vi "OPVM.vi"() -> ()   [LabVIEW 2013]
uses:
  <instrlib>/Keithley 24XX/Public/Data/Read (Multiple Points).vi
  <instrlib>/Keithley 24XX/Keithley 24XX.lvlib
panel:
  out "Voc":sgl
  out "Log IV Graph":cluster{"Voltage":sgl[], "Current":sgl[]}(graph)
  out "IV Graph":cluster{"Voltage":sgl[], "Current":sgl[]}(graph)
  in  "Source Mode  (0: Voltage)":u16(ring) items=["Voltage", "Current"]
  in  "Serial Configuration":T1={"Baud Rate"=9600, "Parity"=0, "Data Bits"=8, "Stop Bits"=10, "Flow Control"=0} {"Flow Control" items=["None", "XON/XOFF", "RTS/CTS", "XON/XOFF & RTS/CTS", "DTR/DSR", "XON/XOFF & DTR/DSR"]; "Stop Bits" items=["1.0"=10, "1.5"=15, "2.0"=20]; "Data Bits" items=["7"=7, "8"=8]; "Parity" items=["None", "Odd", "Even", "Mark", "Space"]; "Baud Rate" items=["300"=300, "600"=600, "1200"=1200, "2400"=2400, "4800"=4800, "9600"=9600, "19200"=19200]}
  in  "VISA resource name":refnum<visa-resource-name>
  in  "Timeout (10000 ms)":i32=10000 format="%#.6g"
  in  "END":dbl=2.0
  in  "START":dbl=1.0
  in  "Number of Points (5)":u32=5
  in  "Current Range (compliance)":dbl=0.1
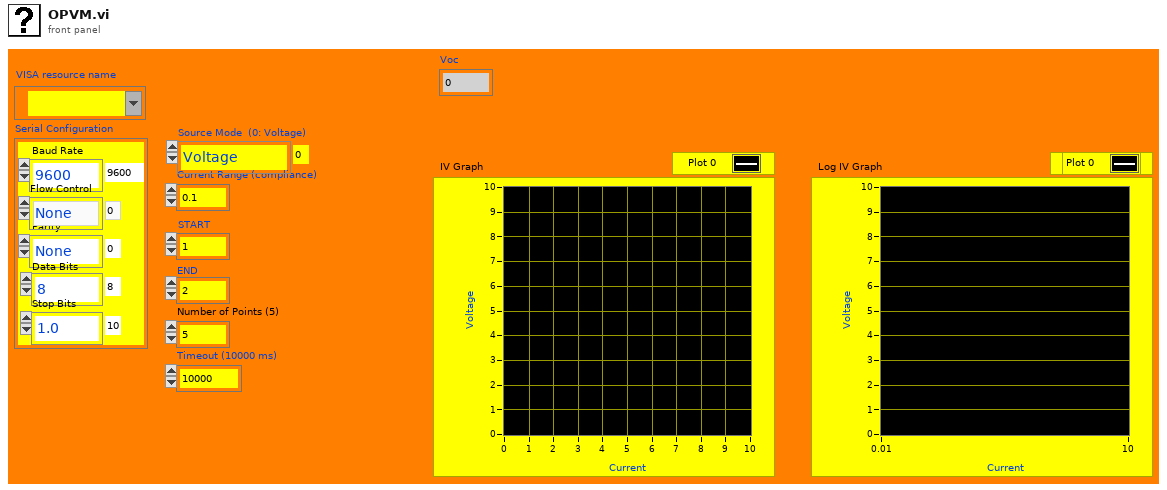
[diagram p1: front panel]
types:
  T1 = cluster{"Baud Rate":u32, "Parity":u16, "Data Bits":u16, "Stop Bits":u16, "Flow Control":u16}
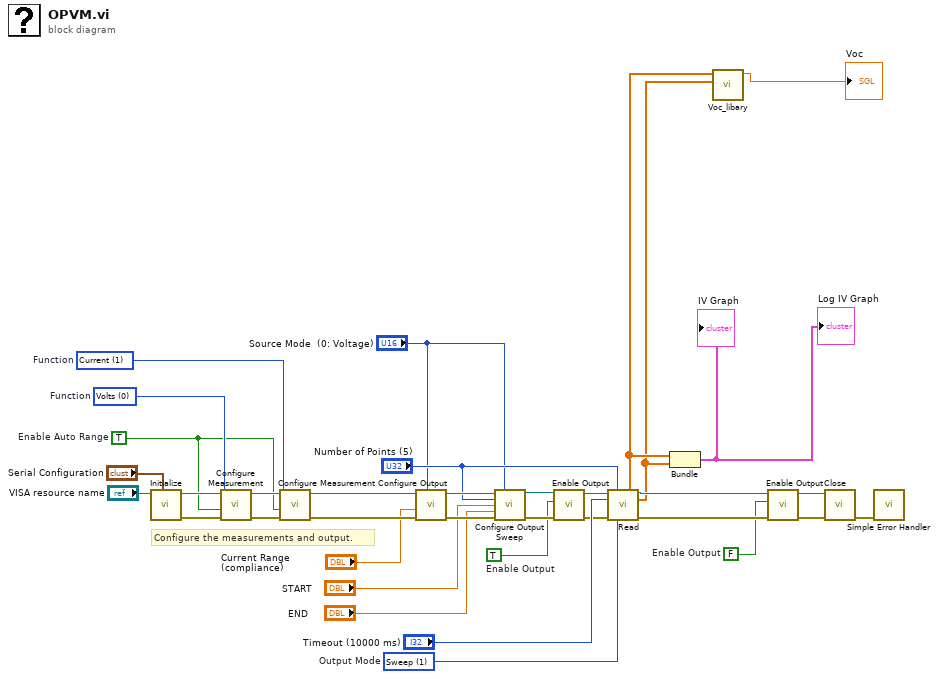
[diagram p0: block diagram]
diagram:
  w6 = TRUE  # Enable Output
  w7 = TRUE  # Enable Auto Range
  w8 = u16 1 items=["Volts", "Current", "Resistance"]  # Function
  w9 = u16 0 items=["Volts", "Current", "Resistance"]  # Function
  w15 = FALSE  # Enable Output
  w21 = u16 1 items=["Fixed", "Sweep", "List"]  # Output Mode
  # "Configure the measurements and output."
  n1 = call <instrlib>:"Initialize.vi"("Serial Configuration"="Serial Configuration", "VISA resource name"="VISA resource name") -> ("error out"=w34:errorcluster, "VISA resource name out"=w35:refnum<visa-resource-name>)  [unwired: 8 in]
  n2 = call <instrlib>:"Configure Measurement.vi"("error in (no error)"=w34, "Enable Auto Range (T:Enable)"=w7, "Function (0: Volts)"=w9, "VISA resource name"=w35) -> ("error out"=w33:errorcluster, "VISA resource name out"=w32:refnum<visa-resource-name>)  [unwired: 6 in]
  n3 = call <instrlib>:"Configure Measurement.vi"("error in (no error)"=w33, "Enable Auto Range (T:Enable)"=w7, "Function (0: Volts)"=w8, "VISA resource name"=w32) -> ("error out"=w30:errorcluster, "VISA resource name out"=w31:refnum<visa-resource-name>)  [unwired: 6 in]
  n4 = call <instrlib>:"Configure Output.vi"("Source Mode  (0: Voltage)"="Source Mode  (0: Voltage)", "error in (no error)"=w30, "Compliance  Level (0.1)"="Current Range (compliance)", "VISA resource name"=w31) -> ("error out"=w29:errorcluster, "VISA resource name out"=w28:refnum<visa-resource-name>)  [unwired: 6 in]
  n5 = call <instrlib>:"Configure Output Sweep.vi"("VISA resource name"=w28, "Source Mode  (0: Voltage)"="Source Mode  (0: Voltage)", "Number of Points (5)"="Number of Points (5)", "Minimum Amplitude (1)"="START", "Maximum Amplitude (2)"="END", "error in (no error)"=w29) -> ("VISA resource name out"=w12:refnum<visa-resource-name>, "error out"=w11:errorcluster)  [unwired: 8 in]
  n6 = call <instrlib>:"Enable Output.vi"("error in (no error)"=w11, "Enable Output (T: Enable)"=w6, "VISA resource name"=w12) -> ("error out"=w14:errorcluster, "VISA resource name out"=w13:refnum<visa-resource-name>)  [unwired: 7 in]
  n7 = call-poly <instrlib>:"Read.vi"("VISA resource name"=w13, "Sample Count (1)"="Number of Points (5)", "Timeout (10000 ms)"="Timeout (10000 ms)", "error in (no error)"=w14, "Output Mode (0: Fixed)"=w21) -> ("Voltage"=w3:sgl[], "VISA resource name out"=w16:refnum<visa-resource-name>, "Current"=w2:sgl[], "error out"=w17:errorcluster)  [unwired: 4 in, 3 out]
  n8 = Bundle("Voltage"=w3, "Current"=w2) -> (→"IV Graph" →"Log IV Graph":cluster{"Voltage":sgl[], "Current":sgl[]})  [unwired: 1 in]
  n9 = call "Voc_libary.vi"("Current"=w2, "Voltage"=w3) -> ("Voc"=→"Voc":sgl)  [unwired: 9 in]
  n10 = call <instrlib>:"Enable Output.vi"("error in (no error)"=w17, "Enable Output (T: Enable)"=w15, "VISA resource name"=w16) -> ("error out"=w18:errorcluster, "VISA resource name out"=w19:refnum<visa-resource-name>)  [unwired: 7 in]
  n11 = call <instrlib>:"Close.vi"("error in (no error)"=w18, "VISA resource name"=w19) -> ("error out"=w20:errorcluster)  [unwired: 9 in]
  n12 = call <vilib>:"Simple Error Handler.vi"("error in (no error)"=w20) -> ()  [unwired: 4 in, 5 out]
